vi "Read Source.vi"(8 "Error In":errorcluster, 11 "Node In":refnum<class "Delimiter.lvclass">) -> (0 "Error Out":errorcluster, 2 "Source":string, 3 "Node Out":refnum<class "Delimiter.lvclass">)   [LabVIEW 2018, in "Toolkit.lvlib" / "Nodes.lvlib" / "Delimiter.lvclass"]
doc: "Gets the original, raw text from the Mustache template that yielded the node during the parsing process."
uses:
  Delimiter.lvclass
  Delimiter.lvclass/Delimiter.ctl
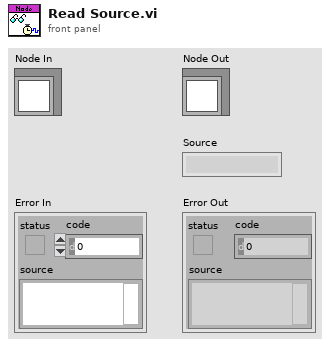
[diagram p1: front panel]
types:
  T1 = typedef "Toolkit.lvlib/Delimiters.ctl" = cluster{"Close":string, "Open":string}
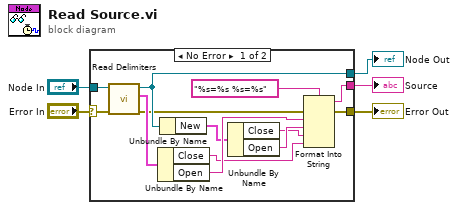
[diagram p0: block diagram]
diagram:
  n1 = case shown="No Error" "Error In" {
    selector: "Error In" -> [w17 w19]
    tunnel: "Node In" -> [w18 w20]
    tunnel: [w16 w20] -> w3
    tunnel: [w7 w19] -> w2
    tunnel: [w6 _] -> w1
    frame No Error {
      n2 = call-dynamic "Read Delimiters.vi"("Error In"=w17, "Node In"=w18) -> ("Error Out"=w8:errorcluster, "Delimiters"=w14:T1, "Node Out"=w16:refnum<class "Delimiter.lvclass">)  [unwired: 7 in]
      n3 = Unbundle By Name(w14) -> ("Close"=w9:string, "Open"=w13:string)
      n4 = Unbundle By Name(w16) -> ("New"=w12:T1)
      n5 = Unbundle By Name(w12) -> ("Close"=w10:string, "Open"=w11:string)
      n6 = Format Into String(format string="%s=%s %s=%s", error in=w8, w13, w11, w10, w9) -> (resulting string=w6:string, error out=w7:errorcluster)  [unwired: 1 in]
    }
    frame Error {
    }
  }
  "Error Out" <- w2
  "Node Out" <- w3
  "Source" <- w1
